vi "Populate Zip File.vi"(8 "error in (no error)":errorcluster, 10 "Source":path=path "examples/Synchronization", 11 "zip file in":i64) -> (0 "error out":errorcluster, 3 "zip file out":i64)   [LabVIEW 2020]
doc: "This VI will zip up a source directory into a Zip file."
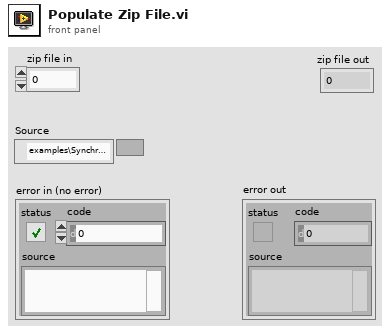
[diagram p1: front panel]
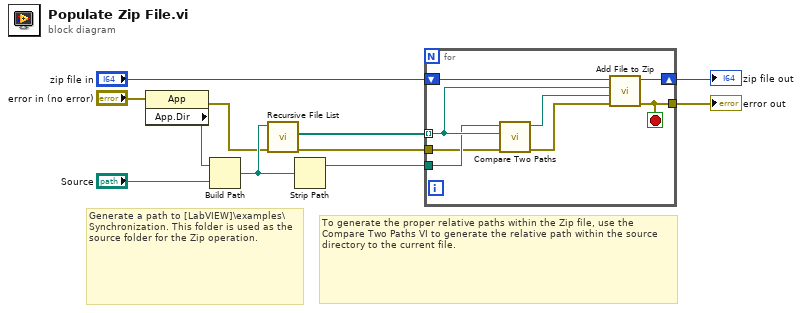
[diagram p0: block diagram]
diagram:
  # "Generate a path to [LabVIEW]\\examples\\Synchronization. This folder is used as the source folder for the Zip operation."
  # "To generate the proper relative paths within the Zip file, use the Compare Two Paths VI to generate the relative path within the source directory to the current file."
  n1 = property class="App"(error in="error in (no error)") -> (error out=w6:errorcluster, "App.Dir"=w9:path)  [unwired: 1 in, 1 out]
  n2 = Build Path(base path=w9, name or relative path="Source") -> (appended path=w8:path)
  n3 = call <vilib>:"Recursive File List.vi"("error in (no error)"=w6, "Folder Path"=w8) -> ("error out"=w3:errorcluster, "All Files in Dir"=w10:path[])  [unwired: 5 in, 3 out]
  n4 = Strip Path(path=w8) -> (stripped path=w5:path)  [unwired: 1 out]
  n5 = for {
    tunnel: w10 -> [w16] mode=indexing
    tunnel: w3 -> [w13]
    tunnel: [w17] -> w1
    shift-right: [w18] -> w11
    shift-left: "zip file in" -> [w19]
    tunnel: w5 -> [w15]
    stop <- w17 stop-if-true
    n6 = call <vilib>:"Compare Two Paths.vi"("error in (no error)"=w13, "Path 2"=w16, "Path 1"=w15) -> ("error out"=w12:errorcluster, "Relative Path from 1 to 2"=w14:path)  [unwired: 5 in, 2 out]
    n7 = call <vilib>:"Add File to Zip.vi"("error in (no error)"=w12, "destination path in zip"=w14, "source file path"=w16, "zip file in"=w19) -> ("error out"=w17:errorcluster, "zip file out"=w18:i64)  [unwired: 6 out]
  }
  "error out" <- w1
  "zip file out" <- w11
